vi "Write Image Name.vi"(8 "error in (no error)":errorcluster, 11 "CCDCamera in":refnum<class "CCDCamera.lvclass">) -> (0 "error out":errorcluster, 3 "CCDCamera out":refnum<class "CCDCamera.lvclass">)   [LabVIEW 2018, in "CCDCamera.lvclass"]
doc: "This VI search for a provided image name on the directiory. If the provided name already existis, the VI adds a numbring to it. If the name does not exists, the VI write it to the class."
uses:
  CCDCamera.lvclass
  CCDCamera.lvclass/CCDCamera.ctl
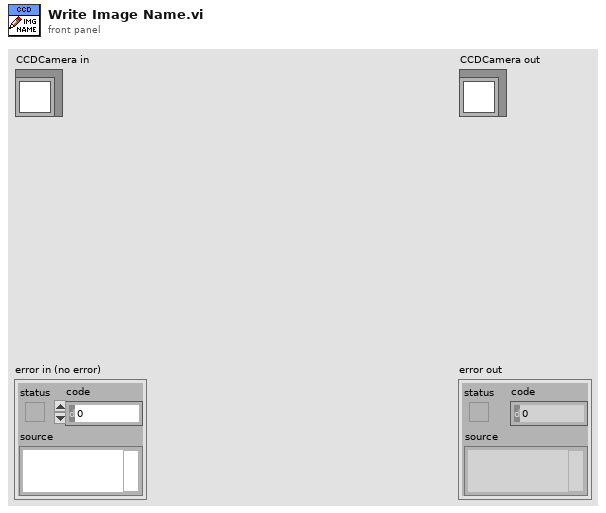
[diagram p1: front panel]
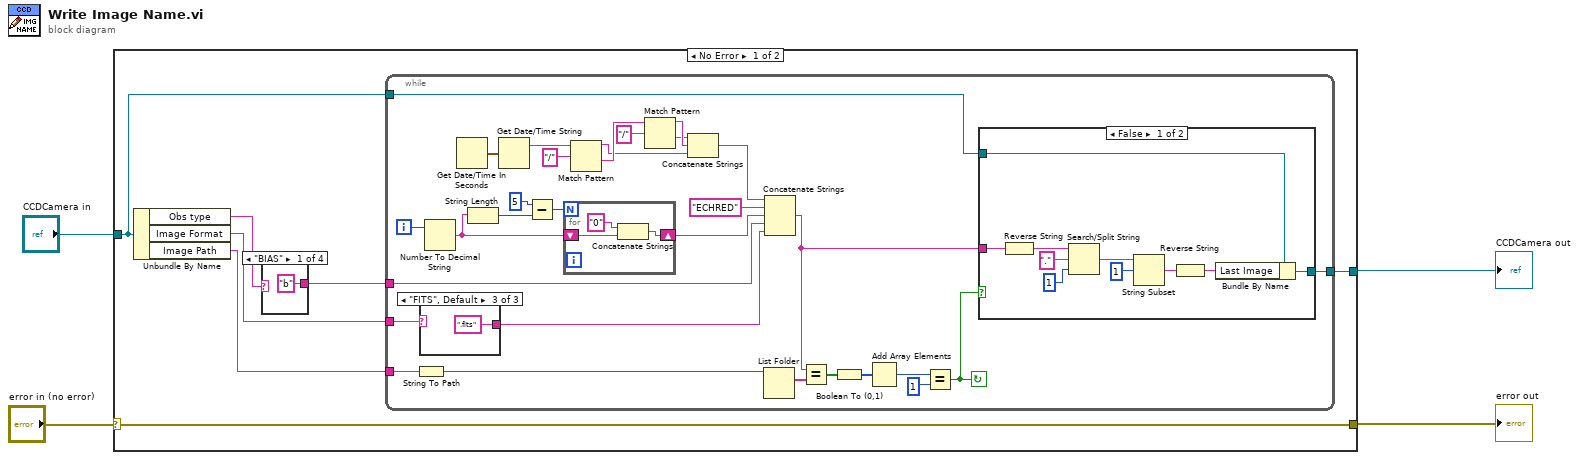
[diagram p0: block diagram]
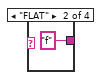
[diagram p2: hidden frame]
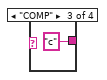
[diagram p3: hidden frame]
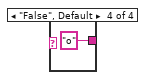
[diagram p4: hidden frame]
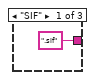
[diagram p5: hidden frame]
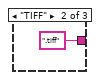
[diagram p6: hidden frame]
diagram:
  n1 = case shown="No Error" "error in (no error)" {
    selector: "error in (no error)" -> [w11 w64]
    tunnel: [w11 w64] -> w3
    tunnel: [w8 w63] -> w1
    tunnel: "CCDCamera in" -> [w9 w63]
    frame No Error {
      n2 = Unbundle By Name(w9) -> ("Obs type"=w6:string, "Image Format"=w7:string, "Image Path"=w10:string)
      n3 = case shown="\"BIAS\"" w6 {
        tunnel: ["b" "f" "c" "o"] -> w5
        frame "BIAS" {
        }
        frame "FLAT" {
        }
        frame "COMP" {
        }
        frame "False", Default {
        }
      }
      n4 = while {
        tunnel: w10 -> [w45]
        tunnel: w9 -> [w38]
        tunnel: [w37] -> w8
        tunnel: w7 -> [w35]
        tunnel: w5 -> [w24]
        i -> [w27]
        stop <- w36 continue-if-true
        n5 = String To Path(string=w45) -> (path=w44:path)
        n6 = case shown="\"FITS\", Default" w35 {
          tunnel: [".sif" ("string") ".tiff" ("string") ".fits" ("string")] -> w25
          frame "SIF" {
          }
          frame "TIFF" {
          }
          frame "FITS", Default {
          }
        }
        n7 = Number To Decimal String(number=w27) -> (decimal integer string=w33:string)  [unwired: 1 in]
        n8 = Get Date/Time In Seconds() -> (seconds since 1Jan1904=w28:timestamp)
        n9 = String Length(string=w33) -> (length=w31:i32)
        n10 = Get Date/Time String(seconds (now)=w28) -> (date string=w17:string)  [unwired: 2 in, 1 out]
        n11 = Subtract(x=5, y=w31) -> (x-y=w30:i32)
        n12 = for {
          N: w30 -> [_]
          shift-right: [w48] -> w34
          shift-left: w33 -> [w46]
          n13 = Concatenate Strings("0" ("string"), w46) -> (w48:string)
        }
        n14 = Match Pattern(string=w17, regular expression="/") -> (before substring=w22:string, after substring=w23:string)  [unwired: 1 in, 2 out]
        n15 = Match Pattern(string=w23, regular expression="/") -> (before substring=w21:string, after substring=w20:string)  [unwired: 1 in, 2 out]
        n16 = Concatenate Strings(w20, w21, w22) -> (w16:string)
        n17 = List Folder(path=w44) -> (filenames=w43:string[])  [unwired: 3 in, 3 out]
        n18 = Concatenate Strings(w16, "ECHRED", w34, w24, w25) -> (w26:string)
        n19 = Equal?(x=w26, y=w43) -> (x = y?=w42:bool[])
        n20 = Boolean To (0,1)(Boolean=w42) -> (0, 1=w41:i16[])
        n21 = Add Array Elements(numeric array=w41) -> (sum=w40:i16)
        n22 = Equal?(x=w40, y=i16 1) -> (x = y?=w36:bool)
        n23 = case shown="False" w36 {
          tunnel: w38 -> [w61 w62]
          tunnel: [w60 w62] -> w37
          tunnel: w26 -> [w59 _]
          frame False {
            n24 = Reverse String(1:w59) -> (0:w56:string)
            n25 = Search/Split String(string=w56, search string/char (-)="." ("regular expression"), offset (0)=1) -> (match + rest of string=w53:string)  [unwired: 2 out]
            n26 = String Subset(string=w53, offset (0)=1) -> (substring=w52:string)  [unwired: 1 in]
            n27 = Reverse String(1:w52) -> (0:w58:string)
            n28 = Bundle By Name(cluster=w61, "Last Image"=w58) -> (w60:refnum<class "CCDCamera.lvclass">)
          }
          frame True {
          }
        }
      }
    }
    frame Error {
    }
  }
  "error out" <- w3
  "CCDCamera out" <- w1
